vi "LWXPS_TZMotorDecouplingMatrixSet.vi"(0 "Value 1 2":dbl, 1 "Value 1 3":dbl, 2 "Value 2 1":dbl, 3 "Value 2 2":dbl, 4 "Value 2 3":dbl, 5 "Value 3 1":dbl, 6 "Value 1 1":dbl, 7 "Value 3 2":dbl, 8 "Group Name":string, 9 "Value 3 3":dbl, 10 "XPS Reference IN":refnum<k24>, 11 "LabVIEW error IN":errorcluster) -> (14 "XPS Reference OUT":refnum<k24>, 15 "Returned error code":i32, 18 "XPS Error String":string, 19 "LabVIEW error OUT":errorcluster)   [LabVIEW 2014]
uses:
  D:/XPSQ8_LabView_Library/Development/Source/Dll/Newport.XPS.CommandInterface.dll
  Dll/Newport.XPS.CommandInterface.dll
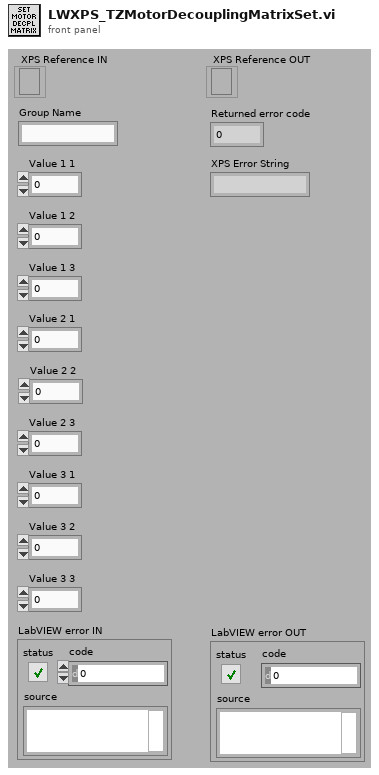
[diagram p1: front panel]
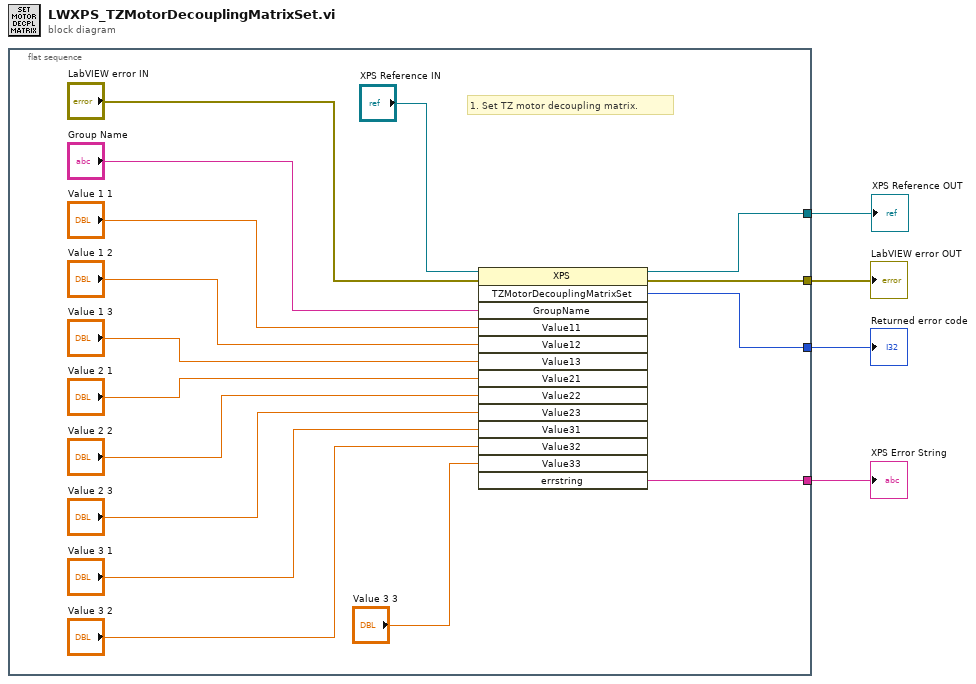
[diagram p0: block diagram]
diagram:
  n1 = flat-sequence {
    tunnel: [w16] -> w4
    tunnel: [w19] -> w3
    tunnel: [w18] -> w2
    tunnel: [w7] -> w1
    frame #0 {
      # "1. Set TZ motor decoupling matrix."
      n2 = invoke class="XPS" method="TZMotorDecouplingMatrixSet"(reference="XPS Reference IN", error in="LabVIEW error IN", "GroupName"="Group Name", "Value11"="Value 1 1", "Value12"="Value 1 2", "Value13"="Value 1 3", "Value21"="Value 2 1", "Value22"="Value 2 2", "Value23"="Value 2 3", "Value31"="Value 3 1", "Value32"="Value 3 2", "Value33"="Value 3 3") -> (reference out=w16:refnum<k24>, error out=w19:errorcluster, "TZMotorDecouplingMatrixSet"=w18:i32, "errstring"=w7:string)  [unwired: 2 in, 10 out]
    }
  }
  "XPS Error String" <- w1
  "XPS Reference OUT" <- w4
  "LabVIEW error OUT" <- w3
  "Returned error code" <- w2
